vi "http get action.vi"(7 "transmit queue":refnum<queue>, 11 "application request in":T1) -> (0 "connection error":errorcluster)   [LabVIEW 2013]
uses:
  http request.ctl
  http method.ctl
  http response.ctl
  http response packet type.ctl
panel:
  in  "other":string
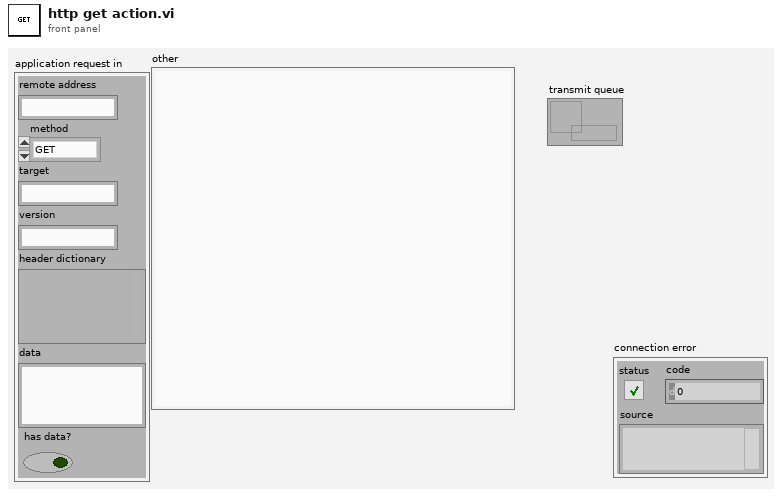
[diagram p1: front panel]
types:
  T1 = typedef "http request.ctl" = cluster{"remote address":string, "method":T2, "target":string, "version":string, "header dictionary":variant, "data":string, "has data?":bool}
  T2 = typedef "http method.ctl" = enum16{"GET", "POST", "PUT", "DELETE", "HEAD", "OPTIONS", "upgrade"}
  T3 = typedef "http response packet type.ctl" = enum16{"full response", "header only", "data only", "last data"}
  T4 = typedef "http response.ctl" = cluster{"packet type":T3, "version":string, "reason code":u16, "status string":string, "header dictionary":variant, "cookies":string[], "data":string}
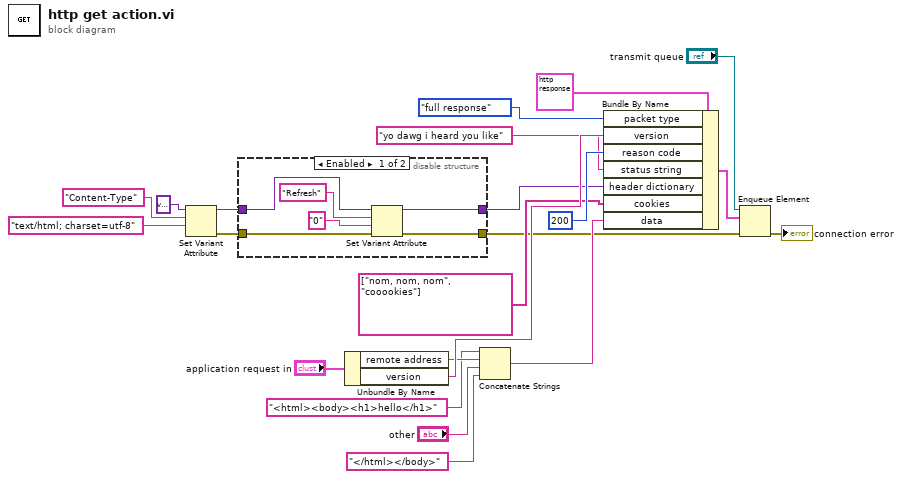
[diagram p0: block diagram]
diagram:
  n1 = Set Variant Attribute(Variant=variant ("variant"), name="Content-Type", value="text/html; charset=utf-8" ("name")) -> (Variant out=w2:variant, error out=w7:errorcluster)  [unwired: 1 in, 1 out]
  n2 = disable-structure shown="Enabled" {
    disable-tunnel: [w28 w30] -> w4
    disable-tunnel: [w27 w29] -> w3
    disable-tunnel: w7 -> [w24 w30]
    disable-tunnel: w2 -> [w23 w29]
    frame Enabled {
      n3 = Set Variant Attribute(Variant=w23, name="Refresh", value="0" ("name"), error in=w24) -> (Variant out=w27:variant, error out=w28:errorcluster)  [unwired: 1 out]
    }
    frame Disabled {
    }
  }
  n4 = Unbundle By Name("application request in") -> ("remote address"=w10:string, "version"=w19:string)
  n5 = Concatenate Strings("<html><body><h1>hello</h1>" ("string"), w10, "other", "</html></body>" ("string")) -> (w11:string)
  n6 = Bundle By Name(cluster=T4 {"packet type"=enum."full response", "version"="", "reason code"=0, "status string"="", "header dictionary"=variant, "cookies"=[], "data"=""} ("application request"), "packet type"=http_response_packet_type."full response", "version"=w19, "reason code"=u16 200, "status string"="yo dawg i heard you like", "header dictionary"=w3, "cookies"=string[] ["nom, nom, nom", "cooookies"], "data"=w11) -> (w5:T4)
  n7 = Enqueue Element(queue="transmit queue", element=w5, error in (no error)=w4) -> (error out=→"connection error":errorcluster)  [unwired: 1 in, 2 out]
